vi "Get All Peaks.vi"(10 "X":dbl[](array[numeric]), 11 "Fit parameters":T1={"Function"=enum."Gauss", "Window width"=nan, "Initial guess"={"Amplitude"=1000.0, "Center"=694.3, "Width"=0.4}} {"Initial guess"."Width" format="%#_gnm"; "Initial guess"."Center" format="%#_gnm"; "Window width" format="%#_6gnm"}) -> (1 "Individual plots":cluster{"X":dbl[], "f(X,a)":dbl[]}[](array[cluster]), 2 "Y":dbl[](array[numeric]))   [LabVIEW 2018]
uses:
  Multi-peak Parameters.ctl
  Peak Parameters.ctl
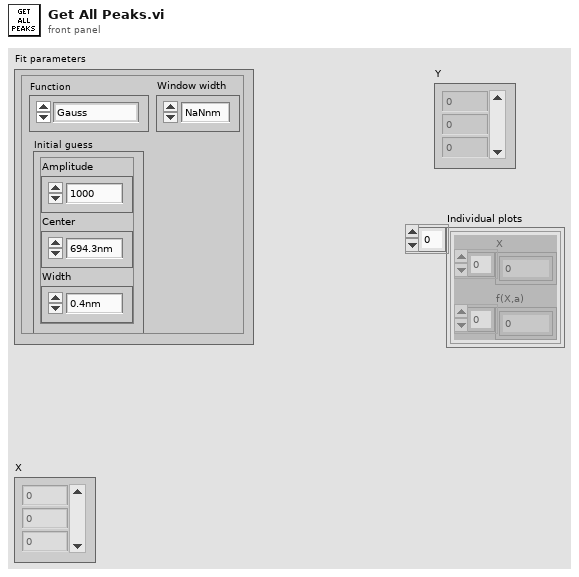
[diagram p1: front panel]
types:
  T1 = typedef "Multi-peak Parameters.ctl" = cluster{"Function":enum16{"Gauss", "Lorentz"}, "Window width":dbl, "Initial guess":T2}
  T2 = typedef "Peak Parameters.ctl" = cluster{"Amplitude":dbl, "Center":dbl, "Width":dbl}
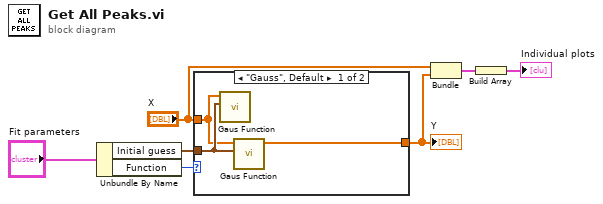
[diagram p0: block diagram]
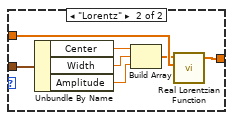
[diagram p2: hidden frame]
diagram:
  n1 = Unbundle By Name("Fit parameters") -> ("Initial guess"=w7:T2, "Function"=w5:enum16{"Gauss", "Lorentz"})
  n2 = case shown="\"Gauss\", Default" w5 {
    tunnel: w7 -> [w10 w14]
    tunnel: "X" -> [w9 w13]
    tunnel: [w8 w11] -> w2
    frame "Gauss", Default {
      n3 = call "Gaus Function.vi"("Fit params"=w10, "X"=w9) -> ()  [unwired: 9 in, 1 out]
      n4 = call "Gaus Function.vi"("Fit params"=w10, "X"=w9) -> ("Y"=w8:dbl[])  [unwired: 9 in]
    }
    frame "Lorentz" {
      n5 = Unbundle By Name(w14) -> ("Center"=w17:dbl, "Width"=w16:dbl, "Amplitude"=w15:dbl)
      n6 = Build Array(w17, w16, w15) -> (w12:dbl[])
      n7 = call "Real Lorentzian Function.vi"("X"=w13, "a"=w12) -> ("f(X,a)"=w11:dbl[])  [unwired: 2 in, 2 out]
    }
  }
  "Y" <- w2
  n8 = Bundle("X"="X", "f(X,a)"=w2) -> (w3:cluster{"X":dbl[], "f(X,a)":dbl[]})  [unwired: 1 in]
  n9 = Build Array(w3) -> (→"Individual plots":cluster{"X":dbl[], "f(X,a)":dbl[]}[])
